vi "Create Default Attributes.vi"(5 "Unique ID":string, 7 "Process Executive Ref":refnum<data-value>, 11 "Stop Tire Shine Foam in":refnum<class "Stop Tire Shine Foam.lvclass">) -> (3 "Stop Tire Shine Foam out":refnum<class "Stop Tire Shine Foam.lvclass">)   [LabVIEW 2019, in "Stop Tire Shine Foam.lvclass"]
uses:
  <vilib>/gpm_packages/@cs/Car-wash/Source/Process Steps/Stop Tire Shine Foam/Stop Tire Shine Foam.lvclass
  <vilib>/gpm_packages/@cs/test-executive/Source/Test Executive/ITestExecutive/ITest Executive.lvclass
  c9dddf1e-e3c4-4992-ad2e-fc4666a85a7b.vi
  <vilib>/Utility/error.llb/Error Cluster From Error Code.vi
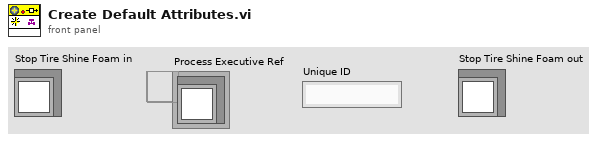
[diagram p1: front panel]
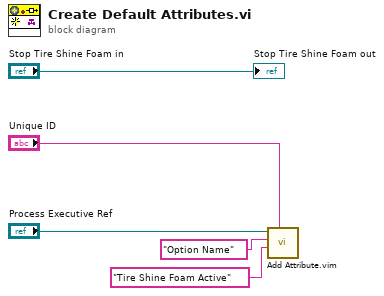
[diagram p0: block diagram]
diagram:
  n1 = call "Add Attribute.vim"("ID"="Unique ID", "Attribute"="Tire Shine Foam Active" ("Item Name"), "Attribute Name"="Option Name" ("Item Name"), "Test Executive Ref"="Process Executive Ref") -> ()  [unwired: 4 in, 4 out]
  "Stop Tire Shine Foam out" <- "Stop Tire Shine Foam in"
